vi "HeaderAction.vi"(0 "InstrClass":refnum<class "ThorKDC101.lvclass"> caption="DNL_LabVIEW Object in", 11 "error in (no error)":errorcluster caption="entrée d'erreur (pas d'erreur)") -> (4 "InstrClassOut":refnum<class "ThorKDC101.lvclass"> caption="DNL_LabVIEW Object out", 6 "DataNames":string[](array[string]), 8 "Instr Name":string, 10 "HeaderString":string, 13 "ArrDisplayNames":string[](array[string]), 14 "DisplayNames":string[](array[string]), 15 "error out":errorcluster caption="sortie d'erreur")   [LabVIEW 2019, in "ThorKDC101.lvclass"]
uses:
  ThorKDC101.lvclass
  C:/Programmes Labview/LabscanV1A/DevicesClass/BaseDevice/BaseDevice.lvclass
  ThorKDC101.lvclass/ThorKDC101.ctl
  <userlib>/GenProg/ReadValByRefBool.vi
  <vilib>/Utility/error.llb/Error Cluster From Error Code.vi
  <vilib>/ErrorRing/Error Ring.xnode
  BaseDevice/BaseDevice.lvclass
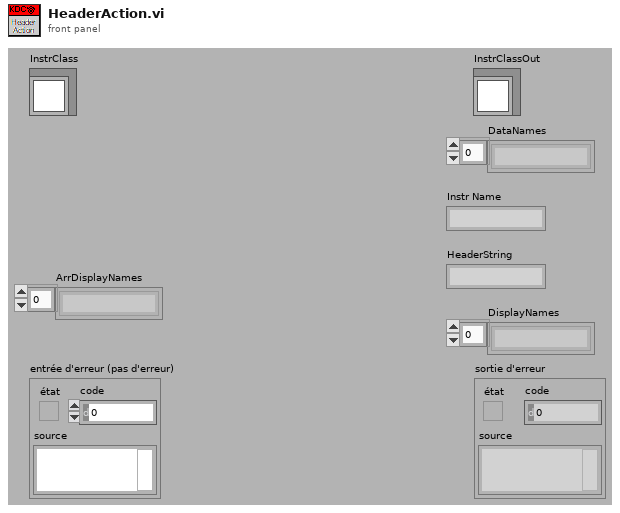
[diagram p1: front panel]
types:
  T1 = typedef "ThorKDC101.lvclass/ThorKDC101_Func.ctl" = enum16{"Position (deg)"}
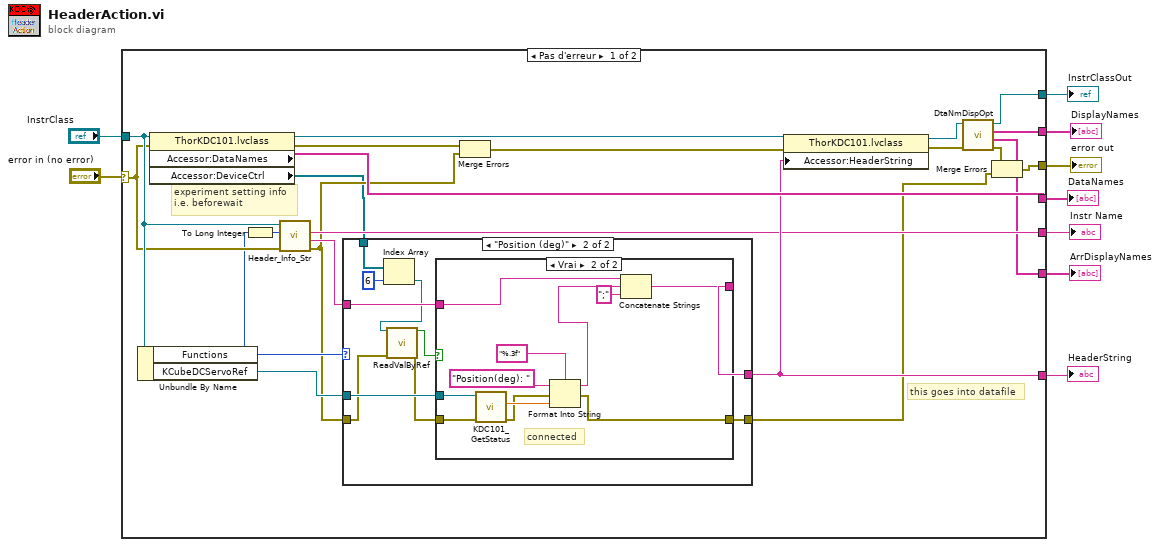
[diagram p0: block diagram]
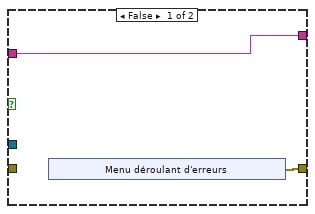
[diagram p3: hidden frame]
diagram:
  n1 = case shown="Pas d'erreur" "error in (no error)" {
    selector: "error in (no error)" -> [w19 w62]
    tunnel: [w28 _] -> w8
    tunnel: [w31 _] -> w7
    tunnel: "InstrClass" -> [w22 w63]
    tunnel: [w11 w62] -> w5
    tunnel: [w25 w63] -> w3
    tunnel: [w21 _] -> w4
    tunnel: [w23 _] -> w2
    tunnel: [w15 _] -> w1
    frame No Error {
      # "this goes into datafile"
      # "experiment setting info\ni.e. beforewait"
      n2 = Unbundle By Name(w22) -> ("Functions"=w17:T1, "KCubeDCServoRef"=w14:refnum<k24>)
      n3 = property class="ThorKDC101.lvclass"(reference=w22, error in=w19) -> (reference out=w30:refnum<class "ThorKDC101.lvclass">, error out=w29:errorcluster, "Accessor:DataNames"=w31:string[], "Accessor:DeviceCtrl"=w12:refnum<vi>[])
      n4 = To Long Integer(number=w17) -> (32bit integer=w16:i32)
      n5 = call-dynamic "Header_Info_Str.vi"("error in (no error)"=w19, "Functions"=w16, "DefaultDev in"=w22) -> ("error out"=w13:errorcluster, "HdrInfoStr"=w20:string, "InstrumentName"=w21:string)  [unwired: 5 in, 1 out]
      n6 = case shown="\"Position (deg)\"" w17 {
        tunnel: [w33 w41] -> w28
        tunnel: w20 -> [w33 w43]
        tunnel: w14 -> [_ w42]
        tunnel: w13 -> [w32 w36]
        tunnel: w12 -> [_ w40]
        tunnel: [w32 w34] -> w10
        frame Default {
        }
        frame "Position (deg)" {
          n7 = Index Array(array=w40, index=6 ("indice")) -> (element=w38:refnum<vi>)
          n8 = call-poly <userlib>:"ReadValByRef.vi"("Control Ref"=w38, "error in"=w36) -> ("Valeur"=w37:bool, "error out"=w35:errorcluster)  [unwired: 12 in]
          n9 = case shown="Vrai" w37 {
            tunnel: w43 -> [w45 w61]
            tunnel: w42 -> [_ w60]
            tunnel: w35 -> [_ w59]
            tunnel: [w45 w52] -> w41
            tunnel: [w44 w51] -> w34
            frame False {
              n10 = xnode "Menu déroulant d'erreurs"() -> ("sortie d'erreur"=w44:errorcluster)
            }
            frame True {
              # "connected"
              n11 = call <userlib>:"KDC101_GetStatus.vi"("error in (no error)"=w59, "KCubeDCServoRef"=w60) -> ("error out"=w53:errorcluster, "ActPos(Deg)"=w58:dbl)  [unwired: 5 in, 3 out]
              n12 = Format Into String(format string="%.3f" ("chaîne de format"), initial string="Position(deg): " ("chaîne initiale"), error in=w53, w58) -> (resulting string=w55:string, error out=w51:errorcluster)
              n13 = Concatenate Strings(w61, w55, ";" ("chaîne")) -> (w52:string)
            }
          }
        }
      }
      n14 = Merge Errors(w29, w13) -> (w18:errorcluster)
      n15 = property class="ThorKDC101.lvclass"(reference=w30, error in=w18, "Accessor:HeaderString"=w28) -> (reference out=w24:refnum<class "ThorKDC101.lvclass">, error out=w27:errorcluster)
      n16 = call "DtaNmDispOpt.vi"("error in (no error)"=w27, "BaseDevice en entrée"=w24) -> ("error out"=w26:errorcluster, "ArrDisplayNames"=w15:string[], "DisplayNames"=w23:string[], "BaseDevice en sortie"=w25:refnum<class "ThorKDC101.lvclass">)  [unwired: 6 in]
      n17 = Merge Errors(w26, w10) -> (w11:errorcluster)
    }
    frame Error {
    }
  }
  "error out" <- w5
  "InstrClassOut" <- w3
  "DataNames" <- w7
  "HeaderString" <- w8
  "Instr Name" <- w4
  "DisplayNames" <- w2
  "ArrDisplayNames" <- w1
